vi "Vent with turbo pump.vi"(8 "error in (no error)":errorcluster) -> (0 "error out":errorcluster)   [LabVIEW 2018]
uses:
  Valve Globals.vi
panel:
  in  "1,2,3,4,5,7,8 open":bool[](array[boolean])=[TRUE, TRUE, TRUE, TRUE, TRUE, FALSE, TRUE, TRUE, FALSE, FALSE, FALSE, FALSE]
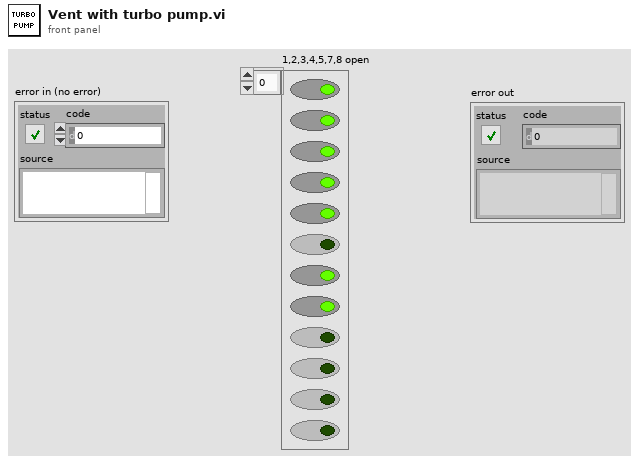
[diagram p1: front panel]
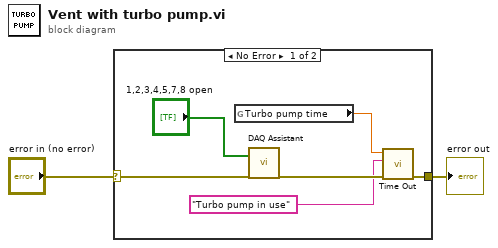
[diagram p0: block diagram]
diagram:
  n1 = case shown="No Error" "error in (no error)" {
    selector: "error in (no error)" -> [w4 w9]
    tunnel: [w5 w9] -> w2
    frame No Error {
      n2 = global read "Valve Globals.vi" "Turbo pump time"() -> (w7:dbl)
      n3 = call "DAQ Assistant"("data"="1,2,3,4,5,7,8 open", "error in"=w4) -> ("error out"=w6:errorcluster)  [unwired: 16 in, 1 out]
      n4 = call "Time Out.vi"("error in (no error)"=w6, 10:"Turbo pump in use", "Numeric"=w7) -> ("error out"=w5:errorcluster)  [unwired: 8 in]
    }
    frame Error {
    }
  }
  "error out" <- w2
